vi "SVX Polar Plot (1 Channel).vi"(0 "magnitudes [RMS]":T9(array[cluster]) {"magnitude" format="%.2f"; "time/rev/RPM" format="%.2f"}, 5 "phases [phase lag]":cluster{"time/rev/RPM":dbl[], "phase":dbl[]}[](array[cluster]) {"phase" format="%.2f"; "time/rev/RPM" format="%.2f"}, 9 "magnitude info":T1={"channel name"="", "description"="", "x-axis units"=0, "spectral info"={"spectrum type"=enum."Power [Magnitude^2]", "linear/dB"=enum."linear", "window"=0, "window size"=0, "FFT size"=0}, "engineering units"=1, "custom label"="", "dB reference [EU]"=0.0, "peak units"=enum."rms", "weighting filter"=0, "spectral density?"=FALSE, "unit label"="", "spectrum skewed?"=FALSE, "complimentary spectrum units"=enum."none"} {"x-axis units" items=["Time (s)"=0, "Frequency-CB (Hz)"=1, "Frequency-CPB (Hz)"=1248, "Frequency-Arbitrary (Hz)"=2357, "Quefrency (s)"=2, "Revolutions (rev)"=3, "Order"=4, "Speed (RPM)"=11, "Speed (rad/s)"=21, "Index"=65535]; "weighting filter" items=["Linear", "A-weighting", "B-weighting", "C-weighting", "ITU-R 468-4", "Dolby", "CCITT", "C-message", "Wb", "Wc", "Wd", "We", "Wf", "Wh", "Wj", "Wk", "Wm", "AES17 20 kHz lowpass", "AES17 40 kHz lowpass", "AES17 20 kHz highpass", "AES17 40 kHz highpass"]; "dB reference [EU]" format="%.2f"; "engineering units" items=["custom..."=0, "V"=1, "A"=21, "C"=30, "pC"=31, "s"=32, "-"=29, "Pa"=2, "N"=20, "g"=3, "m/s^2"=4, "m/s"=5, "m"=6, "mm/s"=12, "mm"=13, "micron/s"=14, "micron"=15, "in/s^2"=7, "in/s"=8, "in"=9, "mil/s"=10, "mil"=11, "rad/s^2"=16, "rad/s"=17, "rad"=18, "deg/s^2"=26, "deg/s"=27, "deg"=28, "RPM"=22, "cycle/s^2"=23, "Hz"=24, "cycle"=25, "strain"=19]; "spectral info"."window" items=["None "=0, "Hanning"=1, "Hamming"=2, "Blackman-Harris"=3, "Exact Blackman"=4, "Blackman"=5, "Flat Top"=6, "4 Term B-Harris "=7, "7 Term B-Harris"=8, "Low Sidelobe"=9, "Force - Exponential"=10, "Gaussian"=62]}, 11 "error in (no error)":errorcluster, 12 "channel properties":T7 {"probe angle [deg]" max=360; "direction" items=["CCW", "CW"]}) -> (3 "unit label":string, 4 "polar plot":T8(array[cluster]), 15 "error out":errorcluster)   [LabVIEW 2017, in "SoundVib_OAVisualization.lvlib"]
doc: "Prepares polar plot data for displaying on a Polar Plot. Use this VI to show magnitude versus phase for a specific order. Wire data to the <B>magnitudes [RMS]</B> and <B>phases [phase lag]</B> inputs to determine the polymorphic instance to use or manually select the instance."
uses:
  <vilib>/addons/Sound and Vibration/Order Analysis/Data Presentation/SoundVib_OAVisualization.lvlib
  <vilib>/addons/Sound and Vibration/Order Analysis/Data Presentation/SubVIs/OAT MCM Channel Property.ctl
  <vilib>/addons/_NISVFA/_Shared subVIs/Controls/svc_Spectrum Info.ctl
  <vilib>/addons/_NISVFA/_Shared subVIs/Controls/svc_X-Axis Units.ctl
  <vilib>/addons/_NISVFA/_Shared subVIs/Controls/svc_Spectrum Type.ctl
  <vilib>/addons/_NISVFA/_Shared subVIs/Controls/svc_Engineering Units Text Ring.ctl
  <vilib>/addons/_NISVFA/_Shared subVIs/Controls/svc_Weighting Filter Text Ring.ctl
  <vilib>/addons/_NISVFA/_Shared subVIs/Controls/svc_Complimentary Spectrum Units.ctl
  <vilib>/addons/_NISVFA/_Spectrum Processing/SVFA Unit Conversion (XY) (1 Ch - M Orders).vi
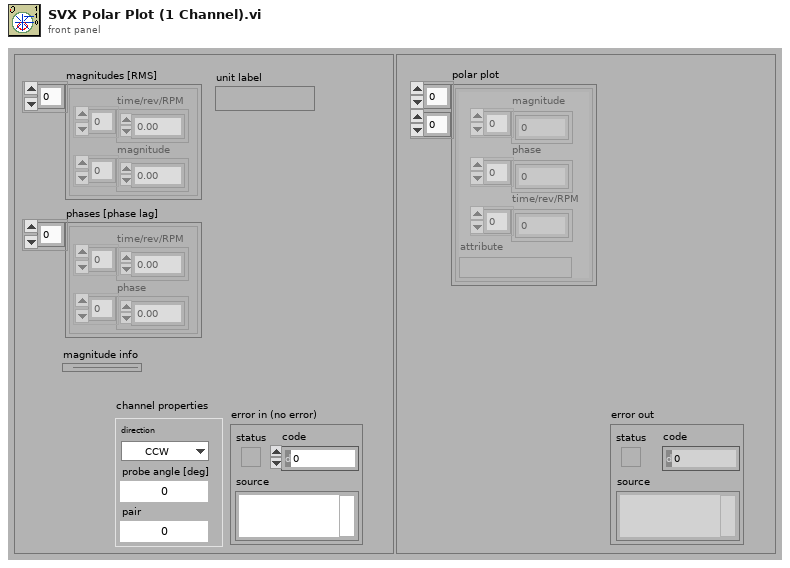
[diagram p1: front panel]
types:
  T1 = typedef "svc_Spectrum Info.ctl" = cluster{"channel name":string, "description":string, "x-axis units":T2, "spectral info":cluster{"spectrum type":T3, "linear/dB":enum16{"linear", "dB"}, "window":u16, "window size":i32, "FFT size":i32}, "engineering units":T4, "custom label":string, "dB reference [EU]":dbl, "peak units":enum16{"rms", "peak", "peak-peak"}, "weighting filter":T5, "spectral density?":bool, "unit label":string, "spectrum skewed?":bool, "complimentary spectrum units":T6}
  T2 = typedef "svc_X-Axis Units.ctl" = u16
  T3 = typedef "svc_Spectrum Type.ctl" = enum16{"FFT Spectrum [complex]", "Amplitude [Magnitude]", "Power [Magnitude^2]", "Cross Spectrum [complex]", "Frequency Response [Complex]"}
  T4 = typedef "svc_Engineering Units Text Ring.ctl" = u16
  T5 = typedef "svc_Weighting Filter Text Ring.ctl" = u16
  T6 = typedef "svc_Complimentary Spectrum Units.ctl" = enum16{"none", "radians", "degrees", "cycles", "imaginary"}
  T7 = typedef "OAT MCM Channel Property.ctl" = cluster{"direction":u16, "probe angle [deg]":u16, "pair":u16}
  T8 = cluster{"magnitude":dbl[], "phase":dbl[], "time/rev/RPM":dbl[], "attribute":variant}[][]
  T9 = cluster{"time/rev/RPM":dbl[], "magnitude":dbl[]}[]
  T10 = cluster{"linear/dB":enum16{"no change", "linear", "dB"}, "dB reference (0: no change)":dbl, "power/magnitude":enum16{"no change", "power", "magnitude"}, "view":enum16{"no change", "rms", "peak", "peak-peak"}}
  T11 = cluster{"magnitude":dbl[], "phase":dbl[], "time/rev/RPM":dbl[], "attribute":variant}
  T12 = cluster{"magnitude":dbl[], "phase":dbl[], "time/rev/RPM":dbl[], "attribute":variant}[]
  T13 = cluster{"time/rev/rpm":dbl[], "magnitude":dbl[]}[]
  T14 = cluster{"dB on? (F)":bool, "unwrap phase? (T)":bool, "unit in degree? (T)":bool}
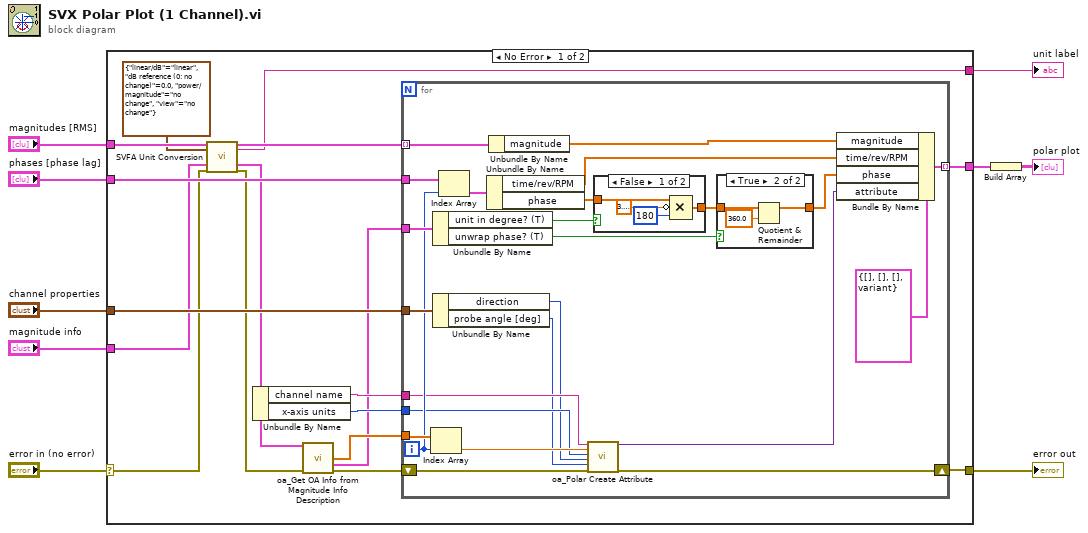
[diagram p0: block diagram]
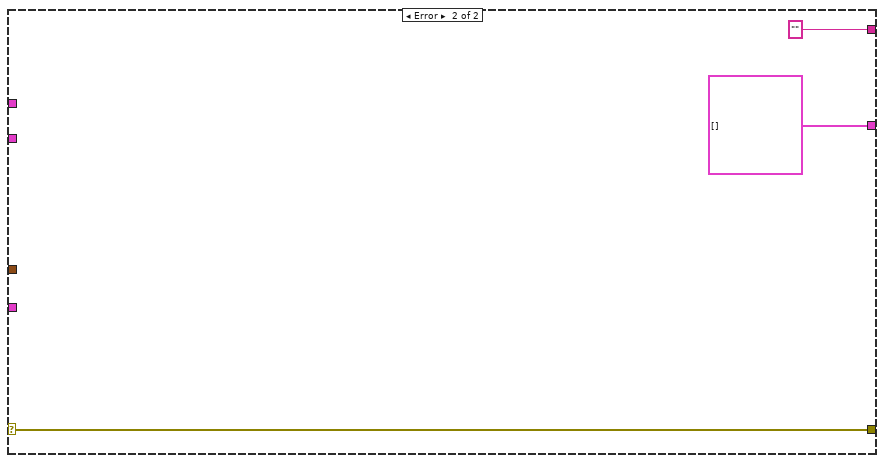
[diagram p4: hidden frame]
diagram:
  n1 = case shown="No Error" "error in (no error)" {
    selector: "error in (no error)" -> [w18 w62]
    tunnel: "magnitudes [RMS]" -> [w21 _]
    tunnel: "phases [phase lag]" -> [w26 _]
    tunnel: "channel properties" -> [w25 _]
    tunnel: [w24 w62] -> w6
    tunnel: [w23 T12 []] -> w2
    tunnel: "magnitude info" -> [w19 _]
    tunnel: [w16 "" ("unit label")] -> w1
    frame No Error {
      n2 = call-poly <vilib>:"SVFA Unit Conversion.vi"("magnitudes"=w21, "desired scaling"=T10 {"linear/dB"=enum."linear", "dB reference (0: no change)"=0.0, "power/magnitude"=enum."no change", "view"=enum."no change"}, "magnitude info in"=w19, "error in (no error)"=w18) -> ("converted magnitudes"=w20:T13, "unit label"=w16:string, "magnitude info out"=w11:T1, "error out"=w12:errorcluster)  [unwired: 12 in]
      n3 = Unbundle By Name(w11) -> ("channel name"=w22:string, "x-axis units"=w15:T2)
      n4 = call <vilib>:"oa_Get OA Info from Magnitude Info Description.vi"("magnitude info"=w11, "error in (no error)"=w12) -> ("orders to compute"=w14:dbl[], "view"=w10:T14, "error out"=w13:errorcluster)  [unwired: 9 in, 2 out]
      n5 = for {
        tunnel: w20 -> [w50] mode=indexing
        tunnel: w26 -> [w44]
        tunnel: w25 -> [w49]
        tunnel: w10 -> [w48]
        tunnel: [w45] -> w23 mode=indexing
        shift-right: [w33] -> w24
        shift-left: w13 -> [w39]
        tunnel: w22 -> [w38]
        tunnel: w14 -> [w42]
        tunnel: w15 -> [w36]
        i -> [w41]
        n6 = Index Array(array=w42, index=w41) -> (element=w37:dbl)
        n7 = Unbundle By Name(w48) -> ("unit in degree? (T)"=w47:bool, "unwrap phase? (T)"=w29:bool)
        n8 = Unbundle By Name(w49) -> ("direction"=w35:u16, "probe angle [deg]"=w34:u16)
        n9 = Index Array(array=w44, index=w41) -> (element=w43:cluster{"time/rev/RPM":dbl[], "phase":dbl[]})
        n10 = Unbundle By Name(w43) -> ("time/rev/RPM"=w31:dbl[], "phase"=w32:dbl[])
        n11 = Unbundle By Name(w50) -> ("magnitude"=w40:dbl[])
        n12 = call <vilib>:"oa_Polar Create Attribute.vi"("channel name"=w38, "order"=w37, "x-axis units"=w36, "rotation direction"=w35, "probe angle [deg]"=w34, "error in (no error)"=w39) -> ("attribute out"=w30:variant, "error out"=w33:errorcluster)  [unwired: 12 in]
        n13 = case shown="False" w47 {
          tunnel: w32 -> [w58 w59]
          tunnel: [w55 w59] -> w28
          frame False {
            n14 = Compound Arithmetic op=MULTIPLY(w58, invert 3.141592653589793, 180) -> (w55:dbl[])
          }
          frame True {
          }
        }
        n15 = case shown="True" w29 {
          tunnel: w28 -> [w51 w54]
          tunnel: [w51 w52] -> w27
          frame False {
          }
          frame True {
            n16 = Quotient & Remainder(x=w54, y=360.0) -> (x-y*floor(x/y)=w52:dbl[])  [unwired: 1 out]
          }
        }
        n17 = Bundle By Name(cluster=T11 {"magnitude"=[], "phase"=[], "time/rev/RPM"=[], "attribute"=variant} ("element"), "magnitude"=w40, "time/rev/RPM"=w31, "phase"=w27, "attribute"=w30) -> (w45:T11)
      }
    }
    frame Error {
    }
  }
  "error out" <- w6
  "unit label" <- w1
  n18 = Build Array(w2) -> (→"polar plot":T8)
